vi "UTIL_Enum COM Ports v1_0_0.vi"(8 "error in":errorcluster) -> (0 "error out":errorcluster, 3 "ports":string[](array[string]))   [LabVIEW 2009]
doc: "UTIL_Enum COM Ports v1_0_0.vi\n\ndll Reads system information and returns an array of usable com ports\n\nCreated 2006 by\nJ. Daren Suntych\nNational Analytics\n970-397-0764"
uses:
  kernel32.dll
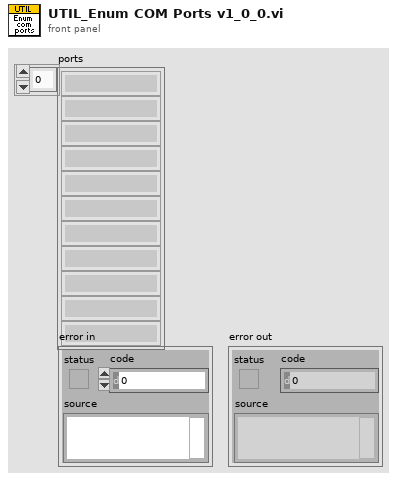
[diagram p1: front panel]
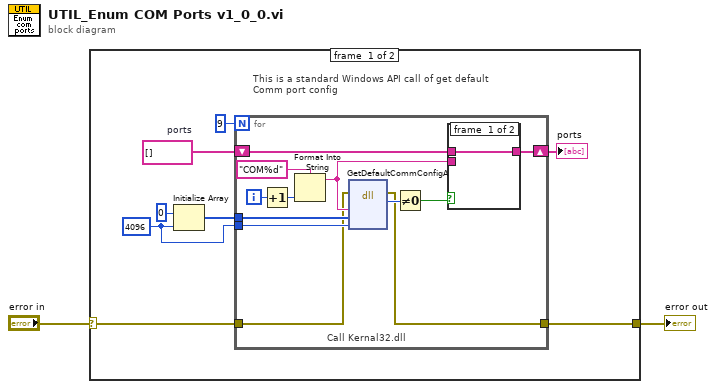
[diagram p0: block diagram]
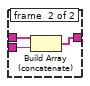
[diagram p2: hidden frame]
diagram:
  n1 = case shown="No Error" "error in" {
    selector: "error in" -> [w3 w27]
    tunnel: [w4 w27] -> w1
    frame #0 {
      w6 = string[] []  # ports
      w8 = u32 4096 ("size")
      # "This is a standard Windows API call of get default\nComm port config"
      n2 = Initialize Array(u8 0 ("size"), w8) -> (w9:u8[])
      n3 = for {
        N: 9 -> [_]
        tunnel: w9 -> [w22]
        tunnel: w8 -> [w21]
        shift-right: [w14] -> w5
        shift-left: w6 -> [w16]
        tunnel: [w11] -> w4
        tunnel: w3 -> [w12]
        i -> [w13]
        # "Call Kernal32.dll"
        n4 = Increment(x=w13) -> (x+1=w20:i32)
        n5 = Format Into String(format string="COM%d" ("Format String"), w20) -> (resulting string=w15:string)  [unwired: 2 in, 1 out]
        n6 = dll-call lib="kernel32.dll" fn="GetDefaultCommConfigA"(error in=w12, "portname"=w15, "pCC"=w22, "size"=w21) -> (error out=w11:errorcluster, w18:i32)  [unwired: 2 in, 4 out]
        n7 = Not Equal To 0?(x=w18) -> (x != 0?=w17:bool)
        n8 = case shown="True" w17 {
          tunnel: w16 -> [w23 w26]
          tunnel: w15 -> [_ w25]
          tunnel: [w23 w24] -> w14
          frame #0 {
          }
          frame #1 {
            n9 = Build Array (concatenate)(w26, w25) -> (w24:string[])
          }
        }
      }
      "ports" <- w5
    }
    frame #1 {
    }
  }
  "error out" <- w1
